vi "Test_WriteValue_InvalidRefnum_Error.vi"(8 "error in (no error)":errorcluster, 11 "TestCase in":refnum<class "TestConfigurationFileBinding.lvclass">) -> (0 "error out":errorcluster, 3 "TestCase out":refnum<class "TestConfigurationFileBinding.lvclass">)   [LabVIEW 2017, in "TestConfigurationFileBinding.lvclass"]
uses:
  TestConfigurationFileBinding.lvclass
  <vilib>/Utility/config.llb/Config Data RefNum.ctl
  Source/Concrete/ConfigurationFileBinding/ConfigurationFileBinding.lvclass/ConfigurationFileBinding.ctl
  Source/Concrete/ConfigurationFileBinding/ConfigurationFileBinding.lvclass
  C:/Git/composed-transport/Source/ITransport/ITransport.lvclass
  <vilib>/Utility/error.llb/Error Cluster From Error Code.vi
  <vilib>/Utility/config.llb/Not A Config Data Refnum.vi
  Source/ITransport/ITransport.lvclass
  <vilib>/Utility/config.llb/NI_LVConfig.lvlib
panel:
  out "Return Error":errorcluster
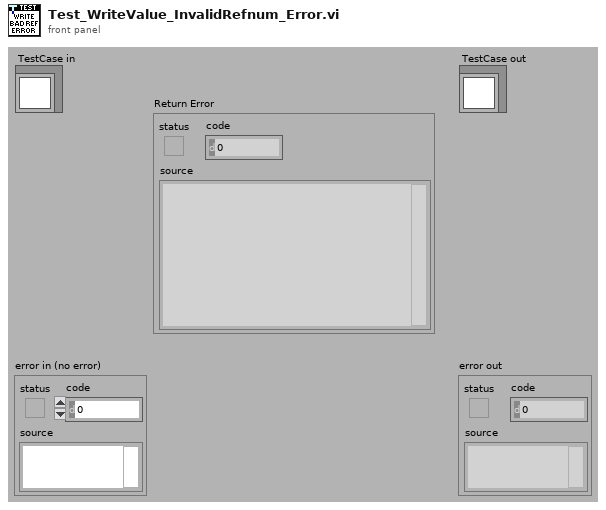
[diagram p1: front panel]
types:
  T1 = typedef "NI_LVConfig.lvlib/Config Data RefNum.ctl" = refnum<k1>
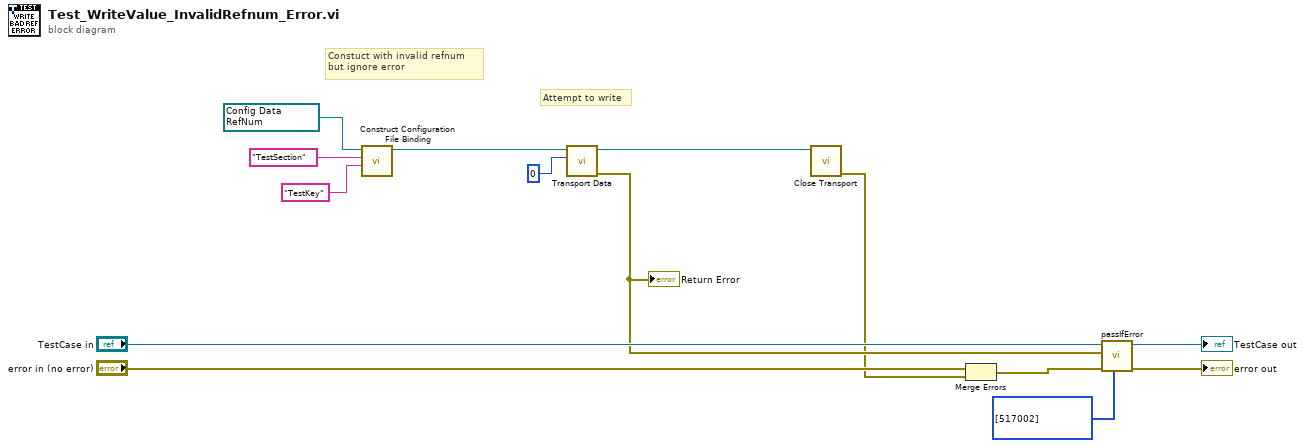
[diagram p0: block diagram]
diagram:
  w2 = T1 refnum items=["config data"] ("Config File Refnum")
  # "Constuct with invalid refnum\nbut ignore error"
  # "Attempt to write"
  n1 = call "Construct Configuration File Binding.vi"("Key Name"="TestKey", "Section Name"="TestSection", "Config File Refnum"=w2) -> ("ConfigurationFileBinding"=w7:refnum<class "ConfigurationFileBinding.lvclass">)  [unwired: 7 in, 1 out]
  n2 = call "Transport Data.vi"("Value"=0, "ITransport in"=w7) -> ("error out"=w5:errorcluster, "ITransport out"=w14:refnum<class "ConfigurationFileBinding.lvclass">)  [unwired: 8 in]
  "Return Error" <- w5
  n3 = call-dynamic "Close Transport.vi"("ITransport in"=w14) -> ("error out"=w4:errorcluster)  [unwired: 10 in]
  n4 = Merge Errors("error in (no error)", w4) -> (w10:errorcluster)
  n5 = call-dynamic "passIfError.vi"("passing error codes (default = any error code)"=i32[] [517002], "error in (no error)"=w10, "error"=w5, "TestCase in"="TestCase in") -> ("error out"=→"error out":errorcluster, "TestCase out"=→"TestCase out":refnum<class "TestConfigurationFileBinding.lvclass">)  [unwired: 6 in]
